vi "Teleop.vi"(10 "Match Info":T1={"Autonomous Elapsed Seconds"=0.0, "TeleOp Elapsed Seconds"=0.0, "Disabled Elapsed Seconds"=0.0, "Visited Autonomous"=FALSE, "Visited TeleOp"=FALSE, "Visited Disabled"=FALSE, "Autonomous Settings"={"Autonomous Style"=enum."Independent", "VI Refnum"=refnum}}, 11 "Call Context":T2) -> ()   [LabVIEW 2016]
doc: "This VI is called for each TeleOp packet received from the DS where the robot is not disabled. It is often used to read from the joysticks and update I/O or to update setpoints for timed control loops. It should complete and return within 20 milliseconds or it may miss DS packets."
uses:
  <vilib>/Rock Robotics/WPI/DriverStation/WPI_DriverStationDerivedRobotMode.ctl
  <vilib>/Rock Robotics/WPI/DriverStation/WPI_DriverStationMatch Info.ctl
  Refname/Controllers.ctl
  Refname/Refname to String (Controllers).vi
  <vilib>/Rock Robotics/WPI/Utilities/WPI_GetSetVariantRefNum.vi
  <vilib>/Rock Robotics/Network Tables/NT Write Boolean.vi
  Robot Global Data.vi
panel:
  out "error out":errorcluster
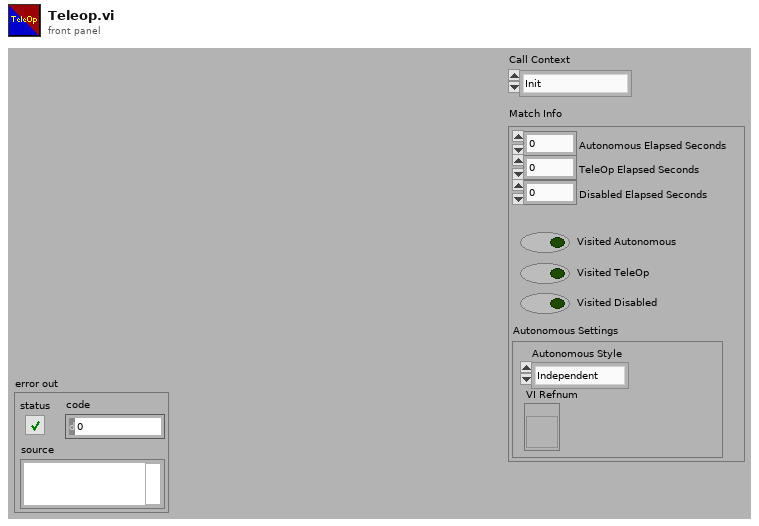
[diagram p1: front panel]
types:
  T1 = typedef "WPI_DriverStationMatch Info.ctl" = cluster{"Autonomous Elapsed Seconds":dbl, "TeleOp Elapsed Seconds":dbl, "Disabled Elapsed Seconds":dbl, "Visited Autonomous":bool, "Visited TeleOp":bool, "Visited Disabled":bool, "Autonomous Settings":cluster{"Autonomous Style":enum16{"Iterative", "Independent"}, "VI Refnum":refnum<vi>}}
  T2 = typedef "WPI_DriverStationDerivedRobotMode.ctl" = enum16{"Init", "Execute", "Stop"}
  T3 = cluster{"X":dbl, "Y":dbl, "Z":dbl, "B (Straight Drive)":bool, "T1 (Climber Up)":bool, "T2 (Climber Down)":bool, "Pinky Trigger (Low Sensitivity Drive)":bool, "Trigger Full Press (Reverse Drive)":bool, "LED Green":bool}
  T4 = typedef "Controllers.ctl" = enum16{"Controller 0", "Controller 1"}
  T5 = typedef "WPI_JoystickDevRef.ctl" = cluster{"Device":T6}
  T6 = typedef "WPI_JoystickDeviceEnum.ctl" = enum16{"USB 0", "USB 1", "USB 2", "USB 3", "USB 4", "USB 5"}
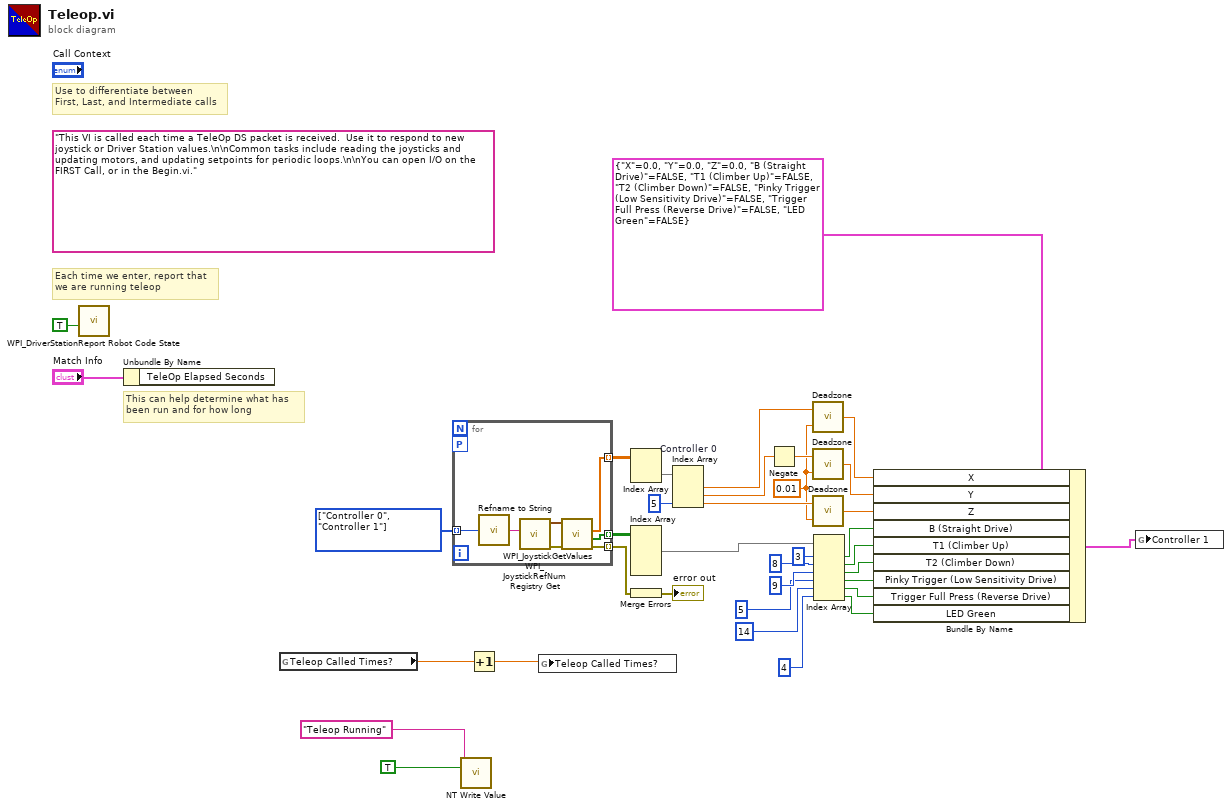
[diagram p0: block diagram]
diagram:
  w23 = 0.01
  w34 = T4[] [enum."Controller 0", enum."Controller 1"] items=["Controller 0", "Controller 1"]
  (unwired) "This VI is called each time a TeleOp DS packet is received.  Use it to respond to new joystick or Driver Station values.\n\nCommon tasks include reading the joysticks and updating motors, and updating setpoints for periodic loops.\n\nYou can open I/O on the FIRST Call, or in the Begin.vi."
  # "Each time we enter, report that\nwe are running teleop"
  # "Use to differentiate between\nFirst, Last, and Intermediate calls"
  # "This can help determine what has\nbeen run and for how long"
  n1 = call <vilib>:"WPI_DriverStationReport Robot Code State.vi"("TeleOp"=TRUE ("Autonomous")) -> ()  [unwired: 10 in, 1 out]
  n2 = Unbundle By Name("Match Info") -> ()  [unwired: 1 out]
  n3 = global read "Robot Global Data.vi" "Teleop Called Times?"() -> (w7:dbl)
  n4 = for {
    tunnel: w34 -> [w43] mode=indexing
    workers-P: _ -> [_]
    tunnel: [w40] -> w33 mode=indexing
    tunnel: [w39] -> w26 mode=indexing
    tunnel: [w37] -> w24 mode=indexing
    n5 = call-poly "Refname to String.vi"("Enum"=w43) -> ("string"=w42:string)
    n6 = call <vilib>:"WPI_JoystickRefNum Registry Get.vi"("refnum name"=w42) -> ("error out"=w38:errorcluster, "JoystickDevRef"=w41:T5)  [unwired: 9 in]
    n7 = call <vilib>:"WPI_JoystickGetValues.vi"("error in (no error)"=w38, "JoystickDevRef"=w41) -> ("error out"=w39:errorcluster, "Buttons"=w37:bool[], "Axes"=w40:dbl[])  [unwired: 5 in, 2 out]
  }
  n8 = call-poly <vilib>:"NT Write Value.vi"("Boolean"=TRUE, "Name"="Teleop Running") -> ()  [unwired: 9 in, 1 out]
  n9 = Increment(x=w7) -> (x+1=w6:dbl)
  n10 = global write "Robot Global Data.vi" "Teleop Called Times?"(w6) -> ()
  n11 = Index Array(array=w33) -> (element=w32:dbl[])  [unwired: 2 in]
  n12 = Index Array(array=w24) -> (element #1=w18:bool[])  [unwired: 4 in, 1 out]
  n13 = Merge Errors(w26) -> (→"error out":errorcluster)
  n14 = Index Array "Controller 0"(array=w32, index #3=5 ("index")) -> (element #1=w30:dbl, element #2=w31:dbl, element #3=w28:dbl)  [unwired: 2 in]
  n15 = Negate(x=w31) -> (-x=w29:dbl)
  n16 = call "Deadzone.vi"("Deadzone"=w23, "Value"=w30) -> ("Numeric"=w20:dbl)
  n17 = call "Deadzone.vi"("Deadzone"=w23, "Value"=w29) -> ("Numeric"=w22:dbl)
  n18 = call "Deadzone.vi"("Deadzone"=w23, "Value"=w28) -> ("Numeric"=w21:dbl)
  n19 = Index Array(array=w18, index #1=3 ("index"), index #2=8 ("index"), index #3=9 ("index"), index #4=5 ("index"), index #5=14 ("index"), index #6=4 ("index")) -> (element #1=w12:bool, element #2=w15:bool, element #3=w14:bool, element #4=w9:bool, element #5=w8:bool, element #6=w1:bool)
  n20 = Bundle By Name(cluster=T3 {"X"=0.0, "Y"=0.0, "Z"=0.0, "B (Straight Drive)"=FALSE, "T1 (Climber Up)"=FALSE, "T2 (Climber Down)"=FALSE, "Pinky Trigger (Low Sensitivity Drive)"=FALSE, "Trigger Full Press (Reverse Drive)"=FALSE, "LED Green"=FALSE} ("input cluster"), "X"=w20, "Y"=w22, "Z"=w21, "B (Straight Drive)"=w12, "T1 (Climber Up)"=w15, "T2 (Climber Down)"=w14, "Pinky Trigger (Low Sensitivity Drive)"=w9, "Trigger Full Press (Reverse Drive)"=w8, "LED Green"=w1) -> (w2:T3)
  n21 = global write "Robot Global Data.vi" "Controller 1"(w2) -> ()
